vi "DriveStraightCommandNavXNew.vi"(6 "Flat Delay":u32, 8 "speed":dbl=0.8, 9 "Fwd Bwd":dbl, 10 "Delay ms":u32=500, 11 "distance":dbl) -> ()   [LabVIEW 2015]
uses:
  Team Code/Robot Global Data.vi
  NavX/navX Library v2/navX Library v2.lvlib
panel:
  out "isFlat":bool
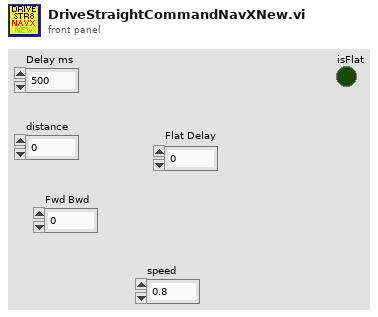
[diagram p1: front panel]
types:
  T1 = enum16{"FlatInitial", "AngleUp", "AngleDown", "FlatFinal"}
  T2 = typedef "WPI_EncoderDevRef.ctl" = cluster{"DevStatus":errorcluster, "EncoderIndex":T3, "CounterIndex":T4, "DistancePerCount":dbl, "Decoding Type":T5}
  T3 = typedef "FPGA_EncoderIdx.ctl" = enum8{"Enc 0", "Enc 1", "Enc 2", "Enc 3", "Enc 4", "Enc 5", "Enc 6", "Enc 7", "Invalid"}
  T4 = typedef "FPGA_CounterCtrSystemIndex.ctl" = enum8{"Ctr 0", "Ctr 1", "Ctr 2", "Ctr 3", "Ctr 4", "Ctr 5", "Ctr 6", "Ctr 7", "Invalid"}
  T5 = typedef "WPI_EncoderType.ctl" = enum16{"1x", "2x", "4x"}
  T6 = typedef "navX Library v2.lvlib/Z900_navX_DeviceTypeDef.ctl" = cluster{"Interface":cluster{"Protocol":T7, "Update Rate (4Hz-60Hz)":u8, "navX Open TypeDef":variant}, "Notify Packet":refnum<notifier>, "Loop VI Refnum":refnum<vi>, "Ready to Close Occurrence Refnum":refnum<k4>}
  T7 = typedef "navX Library v2.lvlib/Z900_navX_ProtocolTypeDef.ctl" = enum16{"SERIAL", "I2C", "SPI"}
  T8 = cluster{"Yaw":dbl, "Roll":dbl, "Pitch":dbl, "Heading":dbl, "Fused Heading":dbl}
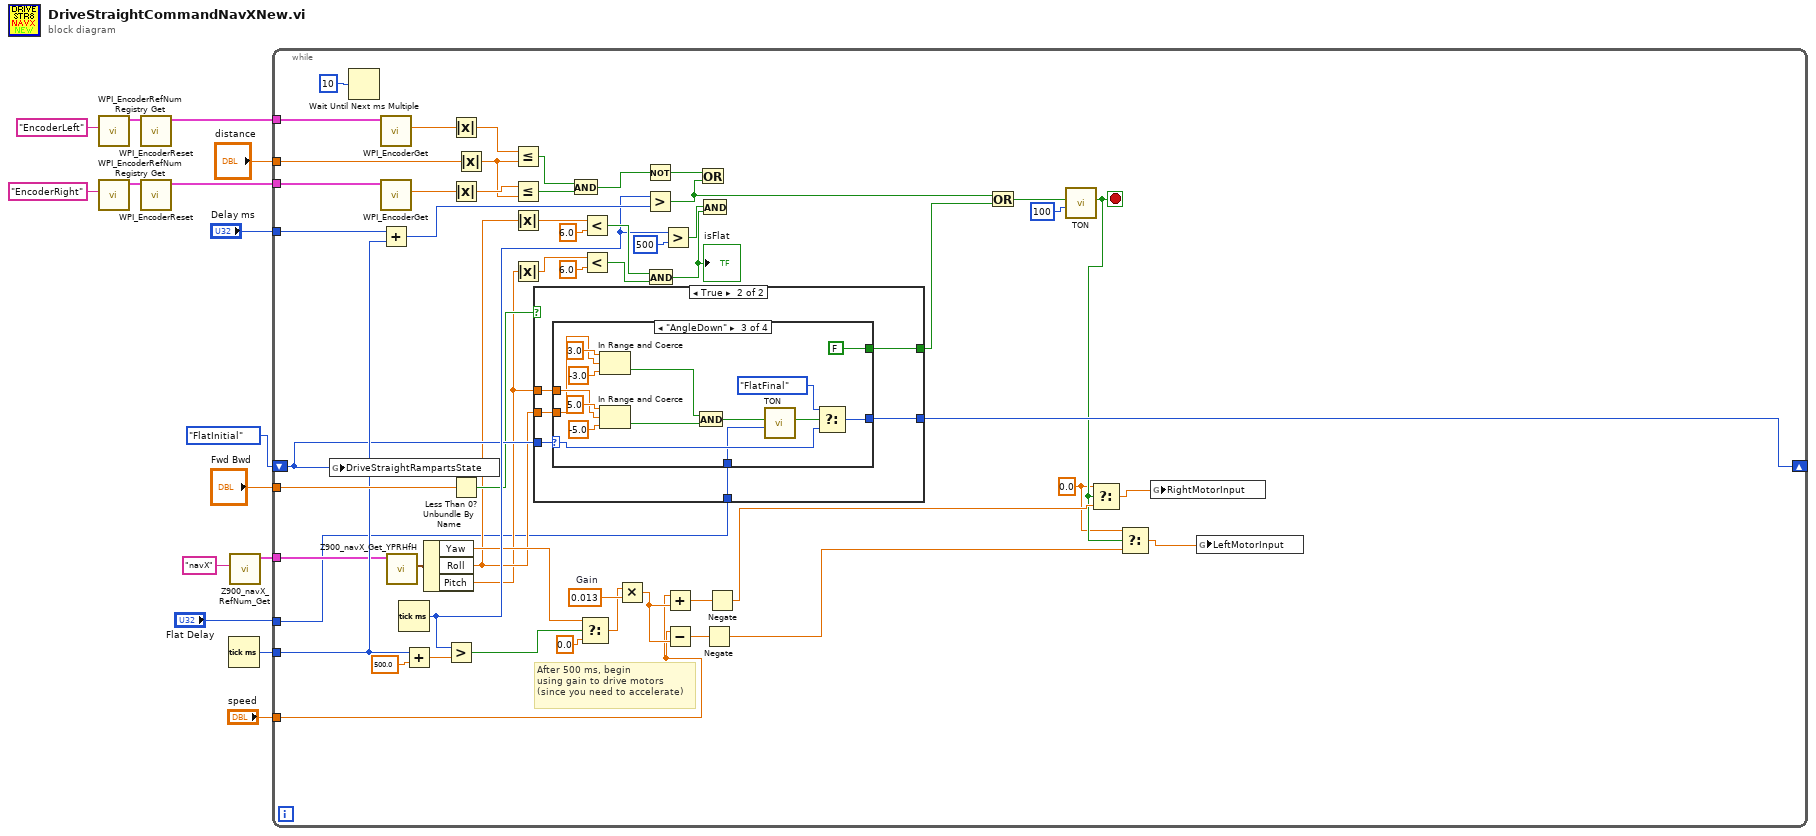
[diagram p0: block diagram]
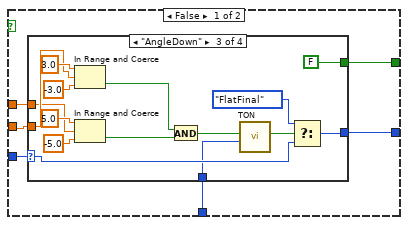
[diagram p2: hidden frame]
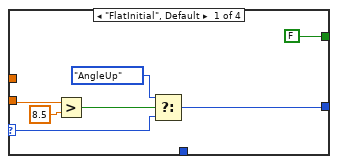
[diagram p3: hidden frame]
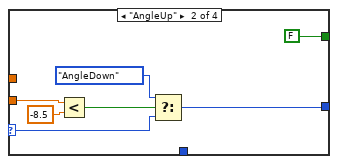
[diagram p4: hidden frame]
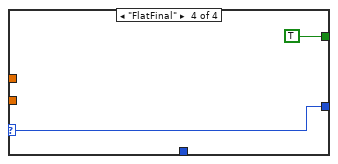
[diagram p5: hidden frame]
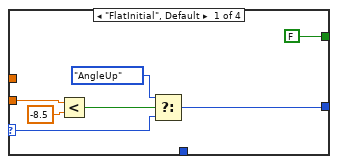
[diagram p6: hidden frame]
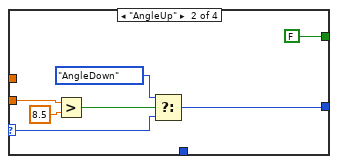
[diagram p7: hidden frame]
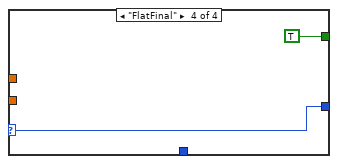
[diagram p8: hidden frame]
diagram:
  n1 = call <vilib>:"WPI_EncoderRefNum Registry Get.vi"("refnum name"="EncoderLeft") -> ("EncoderDevRef"=w14:T2)  [unwired: 9 in, 1 out]
  n2 = call <vilib>:"WPI_EncoderRefNum Registry Get.vi"("refnum name"="EncoderRight") -> ("EncoderDevRef"=w13:T2)  [unwired: 9 in, 1 out]
  n3 = call <vilib>:"WPI_EncoderReset.vi"("EncoderDevRef"=w14) -> ("EncoderDevRef"=w10:T2)  [unwired: 9 in, 1 out]
  n4 = call <vilib>:"WPI_EncoderReset.vi"("EncoderDevRef"=w13) -> ("EncoderDevRef"=w9:T2)  [unwired: 9 in, 1 out]
  n5 = Tick Count (ms)() -> (millisecond timer value=w6:u32)
  n6 = call "Z900_navX_RefNum_Get.vi"("refnum name"="navX") -> ("navX Device"=w4:T6)  [unwired: 9 in, 1 out]
  n7 = while {
    tunnel: "distance" -> [w63]
    tunnel: w10 -> [w66]
    tunnel: w9 -> [w65]
    tunnel: "Fwd Bwd" -> [w64]
    tunnel: "Delay ms" -> [w60]
    tunnel: w6 -> [w58]
    tunnel: w4 -> [w53]
    shift-right: [w41] -> _
    shift-left: T1."FlatInitial" -> [w40]
    tunnel: "speed" -> [w27]
    tunnel: "Flat Delay" -> [w16]
    stop <- w18 stop-if-true
    w17 = 0.0 ("t")
    w33 = 0.013  # Gain
    # "After 500 ms, begin\nusing gain to drive motors\n(since you need to accelerate)"
    n8 = global write "Robot Global Data.vi" "DriveStraightRampartsState"(w40) -> ()
    n9 = Wait Until Next ms Multiple(millisecond multiple=u32 10 ("milliseconds to wait")) -> ()  [unwired: 1 out]
    n10 = call <vilib>:"WPI_EncoderGet.vi"("EncoderDevRef"=w66) -> ("Distance"=w67:dbl)  [unwired: 5 in, 5 out]
    n11 = call <vilib>:"WPI_EncoderGet.vi"("EncoderDevRef"=w65) -> ("Distance"=w68:dbl)  [unwired: 5 in, 5 out]
    n12 = Add(x=w60, y=w58) -> (x+y=w61:u32)
    n13 = call "Z900_navX_Get_YPRHfH.vi"("navX Device"=w53) -> ("YRPHfH"=w52:T8)  [unwired: 7 in, 3 out]
    n14 = Tick Count (ms)() -> (millisecond timer value=w45:u32)
    n15 = Add(x=w58, y=500.0) -> (x+y=w57:dbl)
    n16 = Unbundle By Name(w52) -> ("Yaw"=w31:dbl, "Roll"=w24:dbl, "Pitch"=w23:dbl)
    n17 = Greater?(x=w45, y=w57) -> (0:w29:bool)
    n18 = Absolute Value(x=w67) -> (abs(x)=w69:dbl)
    n19 = Absolute Value(x=w68) -> (abs(x)=w71:dbl)
    n20 = Less Than 0?(x=w64) -> (x < 0?=w34:bool)
    n21 = Absolute Value(x=w63) -> (abs(x)=w70:dbl)
    n22 = Less Or Equal?(x=w69, y=w70) -> (x <= y?=w56:bool)
    n23 = Less Or Equal?(x=w71, y=w70) -> (x <= y?=w55:bool)
    n24 = Absolute Value(x=w24) -> (abs(x)=w51:dbl)
    n25 = Absolute Value(x=w23) -> (abs(x)=w48:dbl)
    n26 = case shown="True" w34 {
      tunnel: [w76 w113] -> w41
      tunnel: w40 -> [w75 w114]
      tunnel: [w77 w112] -> w36
      tunnel: w24 -> [w74 w111]
      tunnel: w23 -> [w73 w110]
      tunnel: w16 -> [w72 w109]
      frame False {
        n27 = case shown="\"AngleDown\"" w75 {
          selector: w75 -> [w84 w91 w101 w108]
          tunnel: [w82 w89 w102 w108] -> w76
          tunnel: [FALSE FALSE FALSE TRUE] -> w77
          tunnel: w74 -> [w78 w85 w94 _]
          tunnel: w73 -> [_ _ w93 _]
          tunnel: w72 -> [_ _ w92 _]
          frame "FlatInitial", Default {
            n28 = Greater?(x=w78, y=8.5) -> (0:w79:bool)
            n29 = Select(t=T1."AngleUp", s=w79, f=w84) -> (s? t:f=w82:T1)
          }
          frame "AngleUp" {
            n30 = Less?(x=w85, y=-8.5) -> (x < y?=w86:bool)
            n31 = Select(t=T1."AngleDown", s=w86, f=w91) -> (s? t:f=w89:T1)
          }
          frame "AngleDown" {
            n32 = In Range and Coerce(upper limit=3.0, x=w94, lower limit=-3.0) -> (In Range?=w97:bool)  [unwired: 1 out]
            n33 = In Range and Coerce(upper limit=5.0, x=w93, lower limit=-5.0) -> (In Range?=w96:bool)  [unwired: 1 out]
            n34 = And(x=w97, y=w96) -> (x .and. y?=w95:bool)
            n35 = call "TON.vi"("Delay (ms)"=w92, "Input"=w95) -> ("Output"=w100:bool)  [unwired: 9 in]
            n36 = Select(t=T1."FlatFinal", s=w100, f=w101) -> (s? t:f=w102:T1)
          }
          frame "FlatFinal" {
          }
        }
      }
      frame True {
        n37 = case shown="\"AngleDown\"" w114 {
          selector: w114 -> [w121 w128 w138 w145]
          tunnel: [w119 w126 w139 w145] -> w113
          tunnel: [FALSE FALSE FALSE TRUE] -> w112
          tunnel: w111 -> [w115 w122 w130 _]
          tunnel: w110 -> [_ _ w131 _]
          tunnel: w109 -> [_ _ w129 _]
          frame "FlatInitial", Default {
            n38 = Less?(x=w115, y=-8.5) -> (x < y?=w116:bool)
            n39 = Select(t=T1."AngleUp", s=w116, f=w121) -> (s? t:f=w119:T1)
          }
          frame "AngleUp" {
            n40 = Greater?(x=w122, y=8.5) -> (0:w123:bool)
            n41 = Select(t=T1."AngleDown", s=w123, f=w128) -> (s? t:f=w126:T1)
          }
          frame "AngleDown" {
            n42 = In Range and Coerce(upper limit=3.0, x=w130, lower limit=-3.0) -> (In Range?=w134:bool)  [unwired: 1 out]
            n43 = In Range and Coerce(upper limit=5.0, x=w131, lower limit=-5.0) -> (In Range?=w133:bool)  [unwired: 1 out]
            n44 = And(x=w134, y=w133) -> (x .and. y?=w132:bool)
            n45 = call "TON.vi"("Delay (ms)"=w129, "Input"=w132) -> ("Output"=w137:bool)  [unwired: 9 in]
            n46 = Select(t=T1."FlatFinal", s=w137, f=w138) -> (s? t:f=w139:T1)
          }
          frame "FlatFinal" {
          }
        }
      }
    }
    n47 = And(x=w56, y=w55) -> (x .and. y?=w39:bool)
    n48 = Select(t=w31, s=w29, f=0.0) -> (s? t:f=w30:dbl)
    n49 = Less?(x=w51, y=6.0) -> (x < y?=w49:bool)
    n50 = Less?(x=w48, y=6.0) -> (x < y?=w46:bool)
    n51 = Multiply(x=w30, y=w33) -> (x*y=w32:dbl)
    n52 = Not(x=w39) -> (.not. x?=w54:bool)
    n53 = Greater?(x=w45, y=w61) -> (0:w37:bool)
    n54 = And(x=w49, y=w46) -> (x .and. y?=w42:bool)
    "isFlat" <- w42
    n55 = Greater?(x=w45, y=u32 500) -> (0:w43:bool)
    n56 = Add(x=w27, y=w32) -> (x+y=w25:dbl)
    n57 = Subtract(x=w27, y=w32) -> (x-y=w26:dbl)
    n58 = Or(x=w54, y=w37) -> ()  [unwired: 1 out]
    n59 = And(x=w43, y=w42) -> ()  [unwired: 1 out]
    n60 = Negate(x=w26) -> (-x=w21:dbl)
    n61 = Negate(x=w25) -> (-x=w22:dbl)
    n62 = Or(x=w37, y=w36) -> (x .or. y?=w35:bool)
    n63 = call "TON.vi"("Delay (ms)"=u32 100, "Input"=w35) -> ("Output"=w18:bool)  [unwired: 9 in]
    n64 = Select(t=w17, s=w18, f=w22) -> (s? t:f=w20:dbl)
    n65 = Select(t=w17, s=w18, f=w21) -> (s? t:f=w19:dbl)
    n66 = global write "Robot Global Data.vi" "RightMotorInput"(w20) -> ()
    n67 = global write "Robot Global Data.vi" "LeftMotorInput"(w19) -> ()
  }
